vi "Trigger Controls with Data from CAT.vi"(5 "West ON/Std OFF":bool, 7 "Mode":enum16{"Run", "Hold", "Off"}(ring)=enum."Off") -> (0 "error out":errorcluster, 3 "Final Output":T2)   [LabVIEW 2012]
uses:
  <vilib>/Platform/TimedLoop/XDataNode/XDataNode.xnode
  <vilib>/Platform/TimedLoop/XDataNode/nitl_modes.ctl
  <vilib>/Platform/TimedLoop/XDataNode/XDNodeRunTimeDep.lvlib
  <vilib>/Platform/TimedLoop/XDataNode/wakeup.ctl
  <vilib>/Platform/TimedLoop/XDataNode/timing_clust.ctl
  Type Defs/Final Output.ctl
  Type Defs/CO2 Settings.ctl
  Type Defs/AD Settings.ctl
  Type Defs/Output Values.ctl
  Type Defs/Output Switches.ctl
  Type Defs/Data Reading.ctl
panel:
  out "Time":string="08:51:17"
  out "Date":string="03/15/13"
  in  "Stop Button":bool
  in  "Tab Control":T1(tab)
  in  "Other Outputs":cluster{"Alarm":bool, "Heater":bool}
  in  "Period mS":i64=1000
  in  "Set Point Alt":dbl=1600.0 min=0.0 max=10000.0 step=1.0
  out "Cycles":i32=3
  out "CO2 ppm":u32(slide)=1231 scale=0.0..10000.0
  out "Alt Dif M":dbl(slide)=204852.9077542369 scale=-1000.0..1000.0 scale format="%.1f"
  out "AD Output":T2
  out "AD State":T2
  out "Data Read":T3={"Date"="03/15/13", "Time"="08:51:25", "CO2- ppm"=1235, "Last Ctrl Word"=4194304, "O2-1 ppm"=2147483648, "O2-2 ppm"=2147483648, "Temp MB"=21.12, "Temp Sensor Module"=23.99, "Press mB"=833.81} {"Last Ctrl Word" format="%.0x"}
  out "Force Output":T4
  out "Force State":T2
  out "Alt Calc":dbl=1449.101900667689
  in  "CO2 Settings":T5={"Run C1"={"A-1,  1"=inf, "A-3,  2"=inf, "A-4, 3"=9000.0, "A-5, 4"=8800.0, "ABCD-7, 5"=9600.0, "A-8, 6"=9200.0, "B-1,  7"=3400.0, "B-3, 8"=3400.0, "B-4,  9"=9000.0, "B-5, 10"=8800.0, "B-8, 11"=9200.0, "C-1, 12"=1800.0, "C-3, 13"=1800.0, "C-4, 14"=9000.0, "C-5,  15"=8800.0, "C-8, 16"=9200.0, "D-1, 17"=inf, "D-3, 18"=3400.0, "D-4,  19"=1800.0, "D-5,  20"=7000.0, "D-8,  21"=9200.0}, "Run C2"={"A-1,  1"=inf, "A-3,  2"=inf, "A-4, 3"=8800.0, "A-5, 4"=8600.0, "ABCD-7, 5"=9600.0, "A-8, 6"=9000.0, "B-1,  7"=3000.0, "B-3, 8"=3000.0, "B-4,  9"=8800.0, "B-5, 10"=8600.0, "B-8, 11"=9000.0, "C-1, 12"=1400.0, "C-3, 13"=1400.0, "C-4, 14"=8800.0, "C-5,  15"=8600.0, "C-8, 16"=9000.0, "D-1, 17"=inf, "D-3, 18"=3000.0, "D-4,  19"=1400.0, "D-5,  20"=6600.0, "D-8,  21"=9000.0}, "Hold C3"={"A-1,  1"=1800.0, "A-3,  2"=1800.0, "A-4, 3"=9000.0, "A-5, 4"=8800.0, "ABCD-7, 5"=9600.0, "A-8, 6"=9200.0, "B-1,  7"=3400.0, "B-3, 8"=3400.0, "B-4,  9"=9000.0, "B-5, 10"=8800.0, "B-8, 11"=9200.0, "C-1, 12"=1800.0, "C-3, 13"=1800.0, "C-4, 14"=9000.0, "C-5,  15"=8800.0, "C-8, 16"=9200.0, "D-1, 17"=1800.0, "D-3, 18"=3400.0, "D-4,  19"=1800.0, "D-5,  20"=7000.0, "D-8,  21"=9200.0}, "Hold C4"={"A-1,  1"=1400.0, "A-3,  2"=1400.0, "A-4, 3"=8800.0, "A-5, 4"=8600.0, "ABCD-7, 5"=9600.0, "A-8, 6"=9000.0, "B-1,  7"=3000.0, "B-3, 8"=3000.0, "B-4,  9"=8800.0, "B-5, 10"=8600.0, "B-8, 11"=9000.0, "C-1, 12"=1400.0, "C-3, 13"=1400.0, "C-4, 14"=8800.0, "C-5,  15"=8600.0, "C-8, 16"=9000.0, "D-1, 17"=1400.0, "D-3, 18"=3000.0, "D-4,  19"=1400.0, "D-5,  20"=6600.0, "D-8,  21"=9000.0}, "High CO2 Forces "={"A-1, 1"=TRUE, "A-3, 2"=TRUE, "A-4, 3"=FALSE, "A-5, 4"=TRUE, "ABCD-7, 5"=FALSE, "A-8, 6"=TRUE, "B-1,  7"=TRUE, "B-3, 8"=TRUE, "B-4, 9"=FALSE, "B-5, 10"=TRUE, "B-8,  11"=TRUE, "C-1, 12"=TRUE, "C-3, 13"=TRUE, "C-4,  14"=FALSE, "C-5,  15"=TRUE, "C-8, 16"=TRUE, "D-1, 17"=TRUE, "D-3, 18"=TRUE, "D-4, 19"=TRUE, "D-5,  20"=TRUE, "D-8,  21"=TRUE}}
  in  "AD Settings":T8={"Set Point Force"={"A-1,  1"=inf, "A-3,  2"=inf, "A-4, 3"=inf, "A-5, 4"=inf, "ABCD-7, 5"=inf, "A-8, 6"=inf, "B-1,  7"=inf, "B-3, 8"=inf, "B-4,  9"=inf, "B-5, 10"=inf, "B-8, 11"=inf, "C-1, 12"=inf, "C-3, 13"=inf, "C-4, 14"=inf, "C-5,  15"=inf, "C-8, 16"=inf, "D-1, 17"=inf, "D-3, 18"=inf, "D-4,  19"=inf, "D-5,  20"=6000.0, "D-8,  21"=inf}, "Run A1"={"A-1,  1"=inf, "A-3,  2"=inf, "A-4, 3"=50.0, "A-5, 4"=0.0, "ABCD-7, 5"=50.0, "A-8, 6"=inf, "B-1,  7"=inf, "B-3, 8"=150.0, "B-4,  9"=60.0, "B-5, 10"=0.0, "B-8, 11"=60.0, "C-1, 12"=15.0, "C-3, 13"=15.0, "C-4, 14"=50.0, "C-5,  15"=inf, "C-8, 16"=60.0, "D-1, 17"=inf, "D-3, 18"=0.0, "D-4,  19"=15.0, "D-5,  20"=0.0, "D-8,  21"=700.0}, "Run A2"={"A-1,  1"=inf, "A-3,  2"=inf, "A-4, 3"=-30.0, "A-5, 4"=-80.0, "ABCD-7, 5"=-30.0, "A-8, 6"=inf, "B-1,  7"=inf, "B-3, 8"=80.0, "B-4,  9"=15.0, "B-5, 10"=-80.0, "B-8, 11"=15.0, "C-1, 12"=-50.0, "C-3, 13"=-50.0, "C-4, 14"=-30.0, "C-5,  15"=inf, "C-8, 16"=15.0, "D-1, 17"=inf, "D-3, 18"=0.0, "D-4,  19"=-50.0, "D-5,  20"=-80.0, "D-8,  21"=650.0}, "Hold A3"={"A-1,  1"=0.0, "A-3,  2"=0.0, "A-4, 3"=50.0, "A-5, 4"=-150.0, "ABCD-7, 5"=50.0, "A-8, 6"=inf, "B-1,  7"=inf, "B-3, 8"=150.0, "B-4,  9"=60.0, "B-5, 10"=-150.0, "B-8, 11"=60.0, "C-1, 12"=-200.0, "C-3, 13"=-200.0, "C-4, 14"=50.0, "C-5,  15"=inf, "C-8, 16"=60.0, "D-1, 17"=0.0, "D-3, 18"=-150.0, "D-4,  19"=-200.0, "D-5,  20"=-200.0, "D-8,  21"=700.0}, "Hold A4"={"A-1,  1"=-150.0, "A-3,  2"=-150.0, "A-4, 3"=-30.0, "A-5, 4"=-250.0, "ABCD-7, 5"=-30.0, "A-8, 6"=inf, "B-1,  7"=inf, "B-3, 8"=80.0, "B-4,  9"=15.0, "B-5, 10"=-250.0, "B-8, 11"=15.0, "C-1, 12"=-300.0, "C-3, 13"=-300.0, "C-4, 14"=-30.0, "C-5,  15"=inf, "C-8, 16"=15.0, "D-1, 17"=-150.0, "D-3, 18"=-250.0, "D-4,  19"=-300.0, "D-5,  20"=-300.0, "D-8,  21"=650.0}, "High AD Diff "={"A-1, 1"=FALSE, "A-3, 2"=FALSE, "A-4, 3"=FALSE, "A-5, 4"=FALSE, "ABCD-7, 5"=FALSE, "A-8, 6"=TRUE, "B-1,  7"=TRUE, "B-3, 8"=FALSE, "B-4, 9"=TRUE, "B-5, 10"=FALSE, "B-8,  11"=TRUE, "C-1, 12"=FALSE, "C-3, 13"=FALSE, "C-4,  14"=FALSE, "C-5,  15"=TRUE, "C-8, 16"=TRUE, "D-1, 17"=FALSE, "D-3, 18"=FALSE, "D-4, 19"=FALSE, "D-5,  20"=FALSE, "D-8,  21"=TRUE}, "Delay S"={"A-1,  1"=30.0, "A-3,  2"=30.0, "A-4, 3"=1.0, "A-5, 4"=30.0, "ABCD-7, 5"=1.0, "A-8, 6"=1.0, "B-1,  7"=1.0, "B-3, 8"=1.0, "B-4,  9"=1.0, "B-5, 10"=30.0, "B-8, 11"=1.0, "C-1, 12"=30.0, "C-3, 13"=30.0, "C-4, 14"=1.0, "C-5,  15"=1.0, "C-8, 16"=1.0, "D-1, 17"=30.0, "D-3, 18"=30.0, "D-4,  19"=30.0, "D-5,  20"=30.0, "D-8,  21"=1.0}}
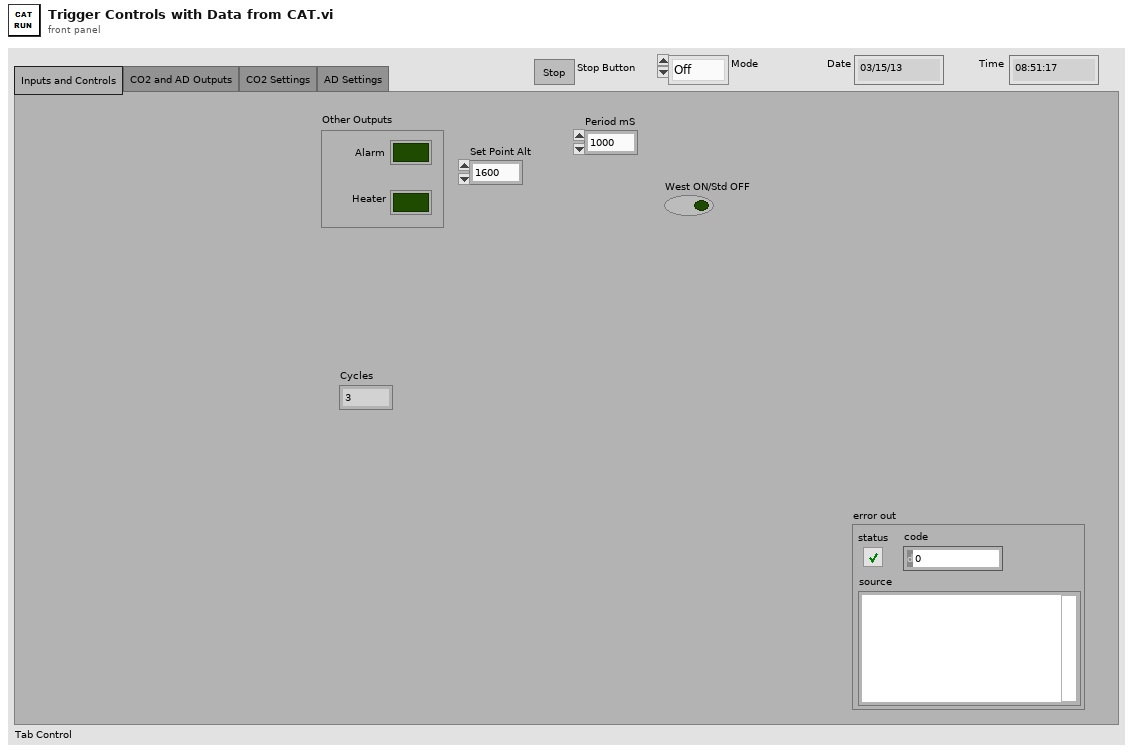
[diagram p1: front panel]
types:
  T1 = enum32{"Inputs and Controls", "CO2 and AD Outputs", "CO2 Settings", "AD Settings"}
  T2 = typedef "Final Output.ctl" = cluster{"Main 1":bool, "Main 2":bool, "Recirc  3":bool, "Scrub 4":bool, "O2 5":bool, "Vent 6":bool, "Boost A 7":bool, "Boost A 8":bool, "Recirc  9":bool, "Scrub 10":bool, "Vent 11":bool, "Boost B 12":bool, "Boost B 13":bool, "Recirc 14":bool, "Scrub 15":bool, "Vent 16":bool, "Main 17":bool, "Boost A 18":bool, "Boost B 19":bool, "Boost F 20":bool, "Vent 2 21":bool}
  T3 = typedef "Data Reading.ctl" = cluster{"Date":string, "Time":string, "CO2- ppm":u32, "Last Ctrl Word":u32, "O2-1 ppm":u32, "O2-2 ppm":u32, "Temp MB":sgl, "Temp Sensor Module":sgl, "Press mB":sgl}
  T4 = cluster{"Main 1":bool, "Main 2":bool, "Recirc  3":bool, "Scrub 4":bool, "O2 5":bool, "Vent 6":bool, "Boost A 7":bool, "Boost A 8":bool, "Recirc  9":bool, "Scrub 10":bool, "Vent 11":bool, "Boost B 12":bool, "Boost B 13":bool, "Recirc 14":bool, "Scrub 15":bool, "Vent 16":bool, "Main 17":bool, "Boost A 18":bool, "Boost B 19":bool, "Boost F 20":bool, "Vent 2 21":bool}
  T5 = typedef "CO2 Settings.ctl" = cluster{"Run C1":T6, "Run C2":T6, "Hold C3":T6, "Hold C4":T6, "High CO2 Forces ":T7}
  T6 = typedef "Output Values.ctl" = cluster{"A-1,  1":dbl, "A-3,  2":dbl, "A-4, 3":dbl, "A-5, 4":dbl, "ABCD-7, 5":dbl, "A-8, 6":dbl, "B-1,  7":dbl, "B-3, 8":dbl, "B-4,  9":dbl, "B-5, 10":dbl, "B-8, 11":dbl, "C-1, 12":dbl, "C-3, 13":dbl, "C-4, 14":dbl, "C-5,  15":dbl, "C-8, 16":dbl, "D-1, 17":dbl, "D-3, 18":dbl, "D-4,  19":dbl, "D-5,  20":dbl, "D-8,  21":dbl}
  T7 = typedef "Output Switches.ctl" = cluster{"A-1, 1":bool, "A-3, 2":bool, "A-4, 3":bool, "A-5, 4":bool, "ABCD-7, 5":bool, "A-8, 6":bool, "B-1,  7":bool, "B-3, 8":bool, "B-4, 9":bool, "B-5, 10":bool, "B-8,  11":bool, "C-1, 12":bool, "C-3, 13":bool, "C-4,  14":bool, "C-5,  15":bool, "C-8, 16":bool, "D-1, 17":bool, "D-3, 18":bool, "D-4, 19":bool, "D-5,  20":bool, "D-8,  21":bool}
  T8 = typedef "AD Settings.ctl" = cluster{"Set Point Force":T6, "Run A1":T6, "Run A2":T6, "Hold A3":T6, "Hold A4":T6, "High AD Diff ":T7, "Delay S":T6}
  T9 = cluster{"Date":string, "Time":string, "CO2- ppm":u32, "Last Ctrl Word":u32, "O2-1 ppm":u32, "O2-2 ppm":u32, "Temp MB":sgl, "Temp Sensor Module":sgl, "Press mB":sgl}
  T10 = cluster{"Main 1":bool, "Main 2":bool, "Recirc  3":bool, "Boost A 7":bool, "Recirc  9":bool, "Scrub 4":bool, "Scrub 10":bool, "O2 5":bool, "Vent 6":bool, "Boost A 8":bool, "Vent 11":bool, "Boost B 12":bool, "Boost B 13":bool, "Recirc 14":bool, "Scrub 15":bool, "Vent 16":bool, "Main 17":bool, "Boost A 18":bool, "Boost B 19":bool, "Boost F 20":bool, "Vent 2 21":bool}
  T11 = typedef "XDNodeRunTimeDep.lvlib/timing_clust.ctl" = cluster{"Expected End [f-1]":u64, "Actual End [f-1]":u64, "Finished Late? [f-1]":bool, "Expected End [i-1]":u64, "Actual End [i-1]":u64, "Finished Late? [i-1]":bool, "Expected Start [i]":u64, "Actual Start [i]":u64, "Expected Start [f]":u64, "Actual Start [f]":u64, "Source Name":string, "Structure Name":string, "Period":i64, "Deadline":i64, "Offset":i64, "Start":i64, "Priority":i32, "Timeout":i32, "Mode":T12, "Wakeup Reason":T13, "Error":errorcluster, "Source Type":string, "Secondary Source Type":string, "Global End Time":u64, "Global Start Time":u64, "Frame Duration":u64, "Iteration Duration":u64, "Assigned CPU":i32, "I/O Scan Engine Mode":u32}
  T12 = typedef "XDNodeRunTimeDep.lvlib/nitl_modes.ctl" = enum32{"No Change", "Process missed periods, maintain original phase", "Discard missed periods, maintain original phase", "Process missed periods, ignore original phase", "Discard missed periods, ignore original phase"}
  T13 = typedef "XDNodeRunTimeDep.lvlib/wakeup.ctl" = enum32{"Normal", "Aborted", "Asynchronous wakeup", "Timing source error", "Timed loop error", "Timeout"}
  T14 = cluster{"A-1,  1":bool, "A-3,  2":bool, "A-4, 3":bool, "A-5, 4":bool, "ABCD-7, 5":bool, "A-8, 6":bool, "B-1,  7":bool, "B-3, 8":bool, "B-4,  9":bool, "B-5, 10":bool, "B-8, 11":bool, "C-1, 12":bool, "C-3, 13":bool, "C-4, 14":bool, "C-5,  15":bool, "C-8, 16":bool, "D-1, 17":bool, "D-3, 18":bool, "D-4,  19":bool, "D-5,  20":bool, "D-8,  21":bool}
  T15 = cluster{bool, bool, bool, bool, bool, bool, bool, bool, bool, bool, bool, bool, bool, bool, bool, bool, bool, bool, bool, bool, bool}
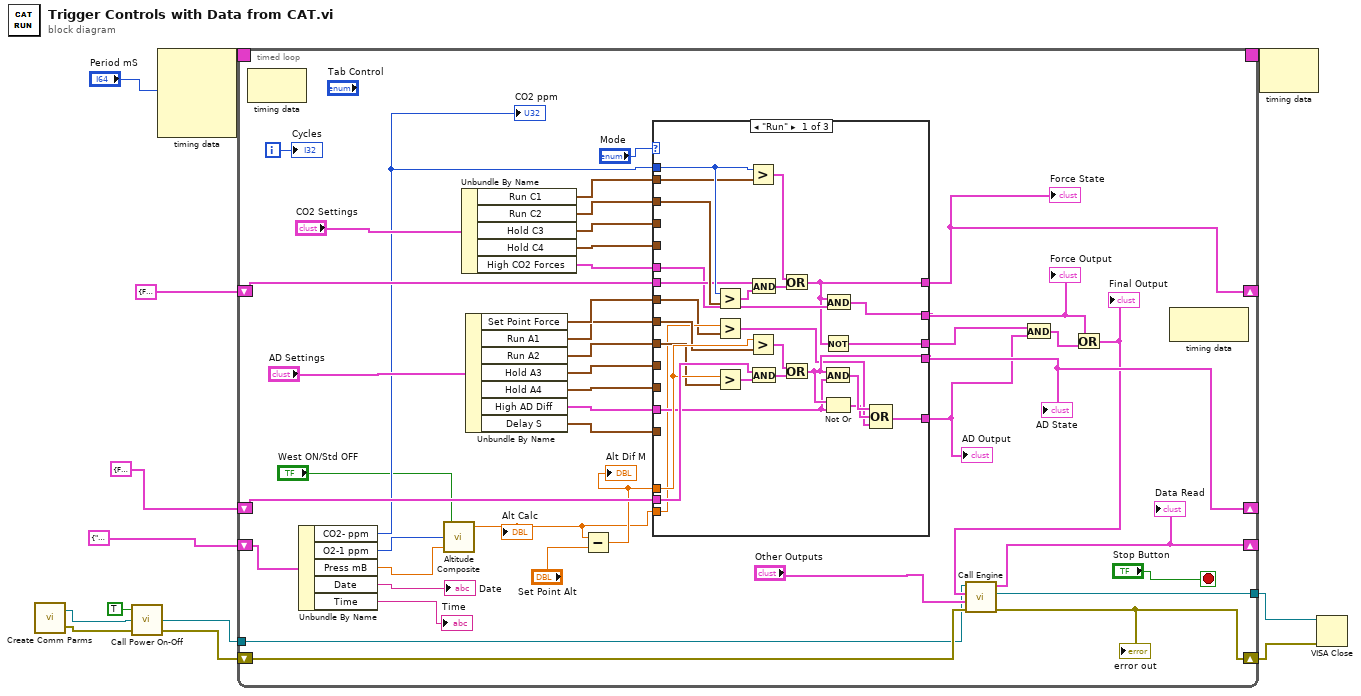
[diagram p0: block diagram]
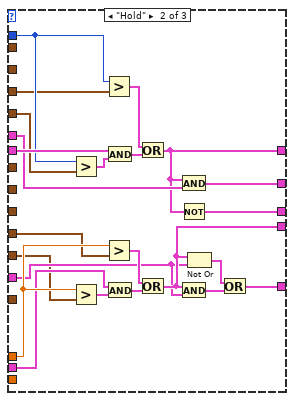
[diagram p2: hidden frame]
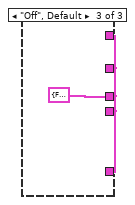
[diagram p3: hidden frame]
diagram:
  n1 = call "Create Comm Parms.vi"() -> ("error out"=w5:errorcluster, "VISA resource name out"=w4:refnum<visa-resource-name>)  [unwired: 2 in]
  n2 = call "Call Power On-Off.vi"("error in"=w5, "VISA resource name"=w4, "On/Off"=TRUE) -> ("error out"=w7:errorcluster, "VISA resource name out"=w1:refnum<visa-resource-name>)  [unwired: 1 in]
  n3 = node-c288("Period mS") -> (w13:T11)  [unwired: 3 in]
  n4 = timed-loop {
    shift-right: [w55] -> _
    shift-left: T10 {"Main 1"=FALSE, "Main 2"=FALSE, "Recirc  3"=FALSE, "Boost A 7"=FALSE, "Recirc  9"=FALSE, "Scrub 4"=FALSE, "Scrub 10"=FALSE, "O2 5"=FALSE, "Vent 6"=FALSE, "Boost A 8"=FALSE, "Vent 11"=FALSE, "Boost B 12"=FALSE, "Boost B 13"=FALSE, "Recirc 14"=FALSE, "Scrub 15"=FALSE, "Vent 16"=FALSE, "Main 17"=FALSE, "Boost A 18"=FALSE, "Boost B 19"=FALSE, "Boost F 20"=FALSE, "Vent 2 21"=FALSE} -> [w54]
    shift-right: [w52] -> _
    shift-left: T10 {"Main 1"=FALSE, "Main 2"=FALSE, "Recirc  3"=FALSE, "Boost A 7"=FALSE, "Recirc  9"=FALSE, "Scrub 4"=FALSE, "Scrub 10"=FALSE, "O2 5"=FALSE, "Vent 6"=FALSE, "Boost A 8"=FALSE, "Vent 11"=FALSE, "Boost B 12"=FALSE, "Boost B 13"=FALSE, "Recirc 14"=FALSE, "Scrub 15"=FALSE, "Vent 16"=FALSE, "Main 17"=FALSE, "Boost A 18"=FALSE, "Boost B 19"=FALSE, "Boost F 20"=FALSE, "Vent 2 21"=FALSE} ("AD State") -> [w51]
    timing: w13 -> [_]
    timing-out: [_] -> w12
    shift-right: [w30] -> w3
    shift-left: w7 -> [w31]
    shift-right: [w27] -> _
    shift-left: T9 {"Date"="", "Time"="", "CO2- ppm"=0, "Last Ctrl Word"=0, "O2-1 ppm"=0, "O2-2 ppm"=0, "Temp MB"=0.0, "Temp Sensor Module"=0.0, "Press mB"=0.0} ("Data Read") -> [w26]
    tunnel: w1 -> [w15]
    tunnel: [w14] -> w2
    i -> [w53]
    stop <- "Stop Button" stop-if-true
    n5 = node-c288() -> ()  [unwired: 1 in, 1 out]
    n6 = Unbundle By Name(w26) -> ("CO2- ppm"=w25:u32, "O2-1 ppm"=w23:u32, "Press mB"=w22:sgl, "Date"=→"Date":string, "Time"=→"Time":string)
    "CO2 ppm" <- w25
    n7 = call "Altitude Composite.vi"("Pressure mBar"=w22, "O2ppm"=w23, "West ON/Std OFF"="West ON/Std OFF") -> ("Alt Eff M 1 correct"=w17:dbl)  [unwired: 2 out]
    "Alt Calc" <- w17
    n8 = Unbundle By Name("CO2 Settings") -> ("Run C1"=w32:T6, "Run C2"=w33:T6, "Hold C3"=w34:T6, "Hold C4"=w35:T6, "High CO2 Forces"=w36:T7)
    n9 = Unbundle By Name("AD Settings") -> ("Set Point Force"=w44:T6, "Run A1"=w43:T6, "Run A2"=w42:T6, "Hold A3"=w41:T6, "Hold A4"=w40:T6, "High AD Diff"=w39:T7, "Delay S"=w38:T6)
    n10 = Subtract(x=w17, y="Set Point Alt") -> (x-y=w21:dbl)
    "Alt Dif M" <- w21
    n11 = case shown="\"Run\"" "Mode" {
      tunnel: w25 -> [w82 w103 _]
      tunnel: w32 -> [w81 _ _]
      tunnel: [w59 w87 w107] -> w55
      tunnel: w33 -> [w83 _ _]
      tunnel: w34 -> [_ w102 _]
      tunnel: w35 -> [_ w101 _]
      tunnel: w54 -> [w78 w104 _]
      tunnel: w36 -> [w60 w93 _]
      tunnel: [w69 w94 w107] -> w50
      tunnel: w21 -> [w74 w98 _]
      tunnel: w43 -> [w73 _ _]
      tunnel: w42 -> [w72 _ _]
      tunnel: w41 -> [_ w85 _]
      tunnel: w40 -> [_ w84 _]
      tunnel: w38 -> [_ _ _]
      tunnel: w39 -> [w67 w91 _]
      tunnel: [w68 w92 w107] -> w52
      tunnel: w51 -> [w75 w97 _]
      tunnel: [w61 w88 w107] -> w49
      tunnel: w17 -> [w64 _ _]
      tunnel: w44 -> [w63 _ _]
      tunnel: [w58 w86 w107] -> w48
      frame "Run" {
        n12 = Greater?(x=w82, y=w83) -> (0:w71:T14)
        n13 = Greater?(x=w64, y=w63) -> (0:w62:T14)
        n14 = Greater?(x=w74, y=w72) -> (0:w70:T14)
        n15 = Greater?(x=w82, y=w81) -> (0:w80:T14)
        n16 = Greater?(x=w74, y=w73) -> (0:w77:T14)
        n17 = And(x=w78, y=w71) -> (x .and. y?=w79:T15)
        n18 = And(x=w75, y=w70) -> (x .and. y?=w76:T15)
        n19 = Or(x=w80, y=w79) -> (x .or. y?=w59:T15)
        n20 = Or(x=w77, y=w76) -> (x .or. y?=w68:T15)
        n21 = Not(x=w59) -> (.not. x?=w58:T15)
        n22 = And(x=w68, y=w67) -> (x .and. y?=w66:T7)
        n23 = Not Or(1:w67, 2:w68) -> (0:w65:T7)
        n24 = And(x=w59, y=w60) -> (x .and. y?=w69:T7)
        n25 = Compound Arithmetic op=OR(w66, w65, w62) -> (w61:T7)
      }
      frame "Hold" {
        n26 = Greater?(x=w103, y=w101) -> (0:w96:T14)
        n27 = Greater?(x=w98, y=w84) -> (0:w95:T14)
        n28 = Greater?(x=w103, y=w102) -> (0:w106:T14)
        n29 = Greater?(x=w98, y=w85) -> (0:w100:T14)
        n30 = And(x=w104, y=w96) -> (x .and. y?=w105:T15)
        n31 = And(x=w97, y=w95) -> (x .and. y?=w99:T15)
        n32 = Or(x=w106, y=w105) -> (x .or. y?=w87:T15)
        n33 = Or(x=w100, y=w99) -> (x .or. y?=w92:T15)
        n34 = And(x=w87, y=w93) -> (x .and. y?=w94:T7)
        n35 = Not(x=w87) -> (.not. x?=w86:T15)
        n36 = And(x=w92, y=w91) -> (x .and. y?=w89:T7)
        n37 = Not Or(1:w91, 2:w92) -> (0:w90:T7)
        n38 = Or(x=w90, y=w89) -> (x .or. y?=w88:T7)
      }
      frame "Off", Default {
        w107 = T10 {"Main 1"=FALSE, "Main 2"=FALSE, "Recirc  3"=FALSE, "Boost A 7"=FALSE, "Recirc  9"=FALSE, "Scrub 4"=FALSE, "Scrub 10"=FALSE, "O2 5"=FALSE, "Vent 6"=FALSE, "Boost A 8"=FALSE, "Vent 11"=FALSE, "Boost B 12"=FALSE, "Boost B 13"=FALSE, "Recirc 14"=FALSE, "Scrub 15"=FALSE, "Vent 16"=FALSE, "Main 17"=FALSE, "Boost A 18"=FALSE, "Boost B 19"=FALSE, "Boost F 20"=FALSE, "Vent 2 21"=FALSE}
      }
    }
    "Force State" <- w55
    "Force Output" <- w50
    "AD State" <- w52
    "AD Output" <- w49
    n39 = And(x=w48, y=w49) -> (x .and. y?=w47:T7)
    n40 = Or(x=w50, y=w47) -> (x .or. y?=w29:T7)
    "Final Output" <- w29
    n41 = call "Call Engine.vi"("error in"=w31, "Other Outputs"="Other Outputs", "Final Output Controls"=w29, "Port"=w15) -> ("error out"=w30:errorcluster, "VISA resource name out"=w14:refnum<visa-resource-name>, "Data Read"=w27:T9)  [unwired: 1 in, 1 out]
    "error out" <- w30
    "Data Read" <- w27
    n42 = node-c288() -> ()  [unwired: 1 in, 1 out]
    "Cycles" <- w53
  }
  n43 = node-c288(w12) -> ()  [unwired: 1 out]
  n44 = VISA Close(VISA resource name=w2, error in (no error)=w3) -> ()  [unwired: 1 out]
